vi "Random Bot Set Coin.vi"(0 "Input Parsed":T1, 11 "error in (no error)":errorcluster) -> (4 "Output Text":string, 15 "error out":errorcluster)   [LabVIEW 2014, in "Dragon Tamers.lvlib"]
uses:
  Typedefs/Input Parsed.ctl
  Typedefs/King.ctl
  Typedefs/Cell Pos.ctl
  Typedefs/Board.ctl
  Typedefs/Board Cell.ctl
  Typedefs/Cell Occupancy.ctl
  Dragon Tamers.lvlib
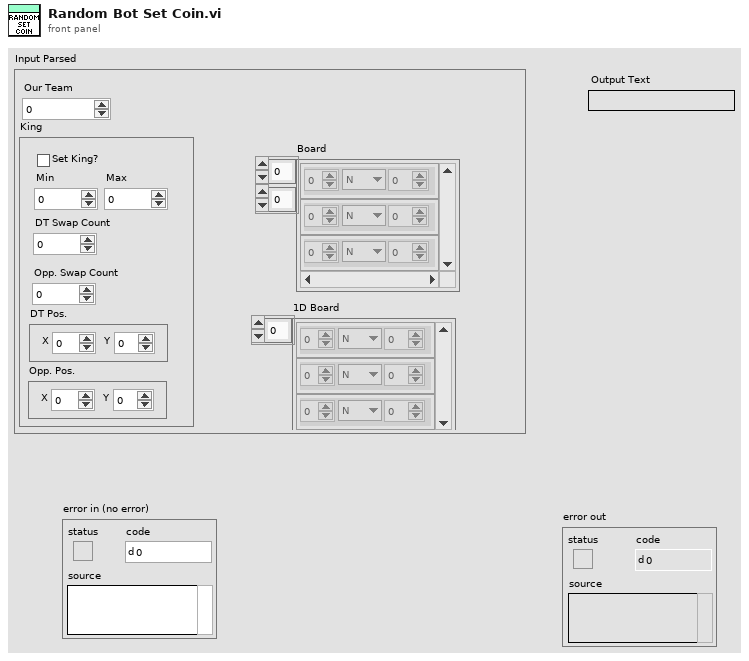
[diagram p1: front panel]
types:
  T1 = typedef "Dragon Tamers.lvlib/Input Parsed.ctl" = cluster{"Our Team":i32, "King":T2, "Board":T4, "1D Board":T5[]}
  T2 = typedef "Dragon Tamers.lvlib/King.ctl" = cluster{"Set King?":bool, "Min":i32, "Max":i32, "DT Swap Count":i32, "Opp. Swap Count":i32, "DT Pos.":T3, "Opp. Pos.":T3}
  T3 = typedef "Dragon Tamers.lvlib/Cell Pos.ctl" = cluster{"X":i32, "Y":i32}
  T4 = typedef "Dragon Tamers.lvlib/Board.ctl" = T5[][]
  T5 = typedef "Dragon Tamers.lvlib/Board Cell.ctl" = cluster{"Team":i32, "Occu.":T6, "Count":i32}
  T6 = typedef "Dragon Tamers.lvlib/Cell Occupancy.ctl" = enum16{"N", "C", "K"}
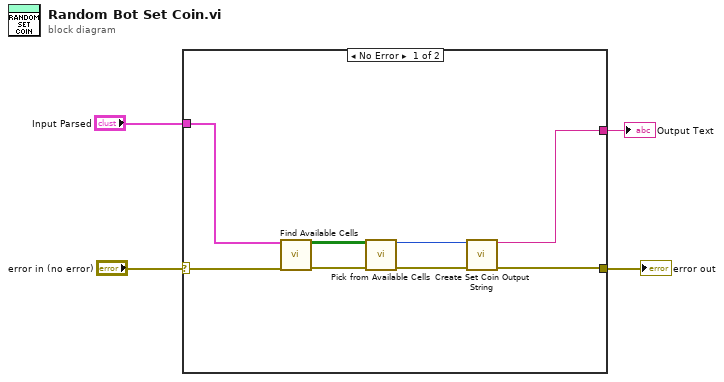
[diagram p0: block diagram]
diagram:
  n1 = case shown="No Error" "error in (no error)" {
    selector: "error in (no error)" -> [w10 w13]
    tunnel: [w7 w13] -> w3
    tunnel: [w5 _] -> w1
    tunnel: "Input Parsed" -> [w9 _]
    frame No Error {
      n2 = call "Find Available Cells.vi"("Input Parsed"=w9, "error in (no error)"=w10) -> ("Board Available"=w11:bool[][], "error out"=w12:errorcluster)  [unwired: 12 in]
      n3 = call "Pick from Available Cells.vi"("Available Cells"=w11, "error in (no error)"=w12) -> ("Picked Cell #"=w6:i32, "error out"=w8:errorcluster)  [unwired: 11 in, 1 out]
      n4 = call "Create Set Coin Output String.vi"("Cell Index"=w6, "error in (no error)"=w8) -> ("Output Text"=w5:string, "error out"=w7:errorcluster)  [unwired: 12 in]
    }
    frame Error {
    }
  }
  "error out" <- w3
  "Output Text" <- w1
